vi "FGV_ReferenceProcess.vi"(7 "Commande":T1, 8 "error in (no error)":errorcluster, 11 "vi reference to add":refnum<vi>) -> (0 "error out":errorcluster, 3 "ProcessReferences":refnum<vi>[](array[refnum]))   [LabVIEW 2013]
uses:
  EnumFgvReferenceProcess.ctl
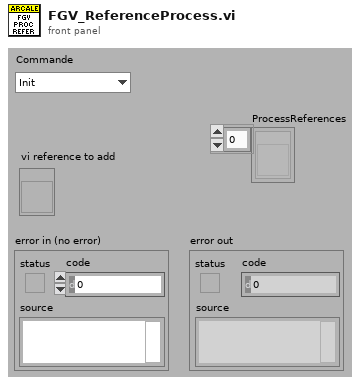
[diagram p1: front panel]
types:
  T1 = typedef "EnumFgvReferenceProcess.ctl" = enum16{"Init", "Get", "Add Reference", "Close References"}
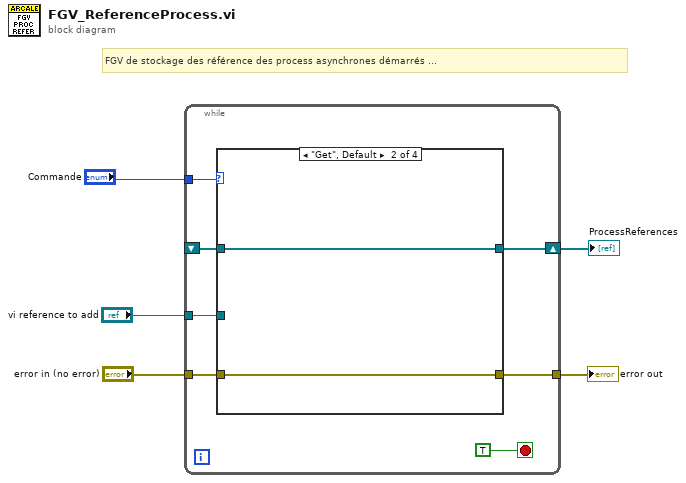
[diagram p0: block diagram]
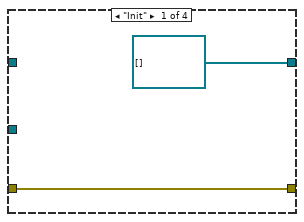
[diagram p2: hidden frame]
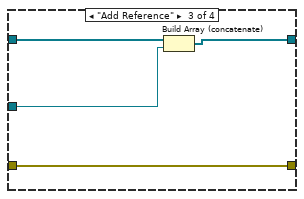
[diagram p3: hidden frame]
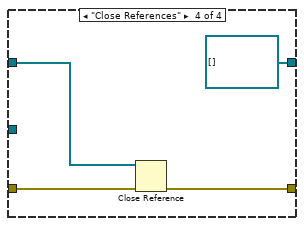
[diagram p4: hidden frame]
diagram:
  # "FGV de stockage des référence des process asynchrones démarrés ..."
  n1 = while {
    tunnel: "Commande" -> [w11]
    tunnel: "vi reference to add" -> [w10]
    shift-right: [w7] -> w5
    shift-left: _ -> [w9]
    tunnel: "error in (no error)" -> [w8]
    tunnel: [w6] -> w4
    stop <- TRUE stop-if-true
    n2 = case shown="\"Get\", Default" w11 {
      tunnel: w10 -> [_ _ w18 _]
      tunnel: w9 -> [_ w15 w20 w24]
      tunnel: w8 -> [w13 w16 w17 w22]
      tunnel: [refnum<vi>[] [] w15 w19 refnum<vi>[] []] -> w7
      tunnel: [w13 w16 w17 w21] -> w6
      frame "Init" {
      }
      frame "Get", Default {
      }
      frame "Add Reference" {
        n3 = Build Array (concatenate)(w20, w18) -> (w19:refnum<vi>[])
      }
      frame "Close References" {
        n4 = Close Reference(reference=w24, error in (no error)=w22) -> (error out=w21:errorcluster)
      }
    }
  }
  "error out" <- w4
  "ProcessReferences" <- w5
